vi "DLIbufferedRead.vi"(9 "timeout(ms)":i32, 10 "Ch.":i32, 11 "URL":string) -> (0 "error out":errorcluster, 1 "state(1or0)":i16, 2 "body":string, 3 "headers":string)   [LabVIEW 2018]
uses:
  DLIbufferState.ctl
  ADAM Client/Sub VIs/ADAM Controls/Remember_value_mode.ctl
  <vilib>/httpClient/LabVIEWHTTPClient.lvlib
panel:
  out "AuditTrail":T1[](array[typedef])
  out "allChs":u32 format="%08b"
  out "age(s)":dbl
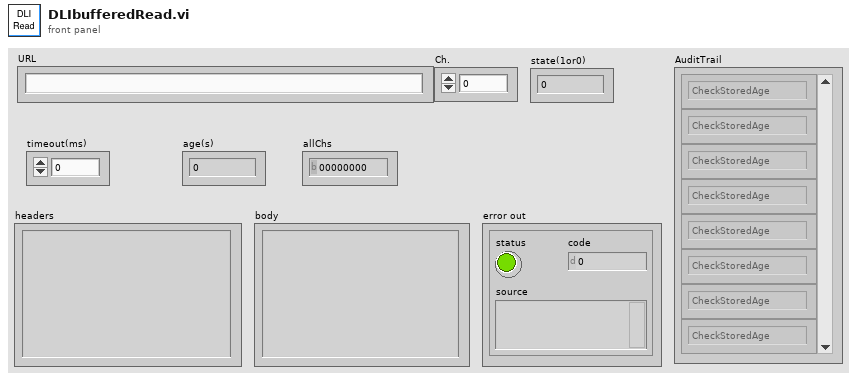
[diagram p1: front panel]
types:
  T1 = typedef "DLIbufferState.ctl" = enum16{"CheckStoredAge", "UseStoredValue", "Read", "Store"}
  T2 = typedef "Remember_value_mode.ctl" = enum16{"Read only", "Read and Write"}
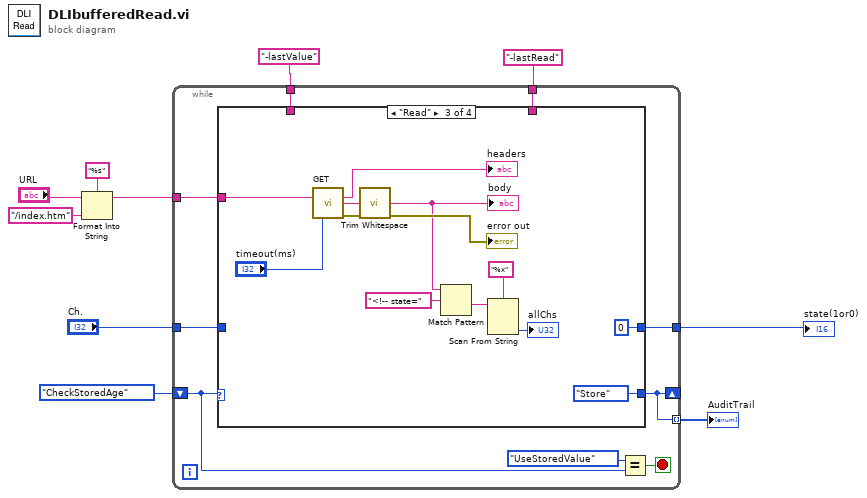
[diagram p0: block diagram]
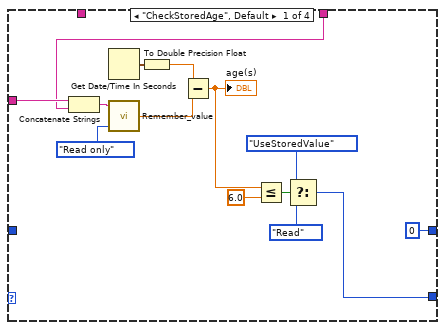
[diagram p2: hidden frame]
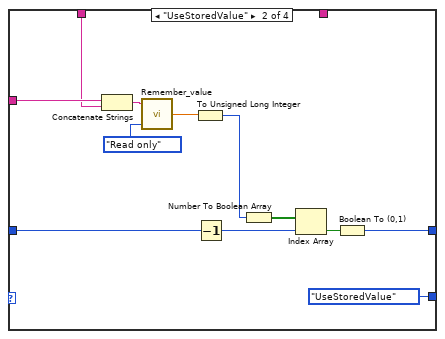
[diagram p3: hidden frame]
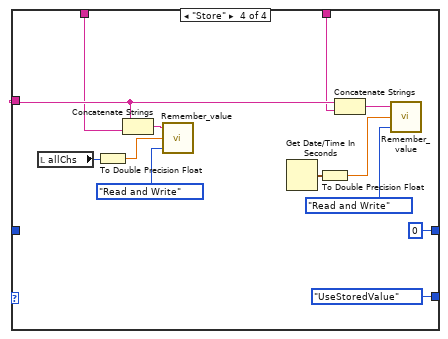
[diagram p4: hidden frame]
diagram:
  n1 = Format Into String(format string="%s", initial string="URL", "/index.htm" ("input 1")) -> (resulting string=w6:string)  [unwired: 1 in, 1 out]
  n2 = while {
    shift-right: [w11] -> _
    shift-left: DLIbufferState."CheckStoredAge" -> [w12]
    tunnel: w6 -> [w19]
    tunnel: "Ch." -> [w18]
    tunnel: [w17] -> w4
    tunnel: "-lastRead" ("string") -> [w16]
    tunnel: "-lastValue" ("string") -> [w15]
    tunnel: [w11] -> w1 mode=indexing
    stop <- w14 stop-if-true
    n3 = case shown="\"Read\"" w12 {
      tunnel: w19 -> [w30 w43 w50 w64]
      tunnel: w18 -> [_ w37 _ _]
      tunnel: [i16 0 w36 i16 0 i16 0] -> w17
      tunnel: [w23 DLIbufferState."UseStoredValue" DLIbufferState."Store" DLIbufferState."UseStoredValue"] -> w11
      tunnel: w16 -> [w20 _ _ w61]
      tunnel: w15 -> [_ w35 _ w60]
      frame "CheckStoredAge", Default {
        n4 = Concatenate Strings(w30, w20) -> (w31:string)
        n5 = Get Date/Time In Seconds() -> (seconds since 1Jan1904=w33:timestamp)
        n6 = call "Remember_value.vi"("Mode"=Remember_value_mode."Read only", "Ch name"=w31) -> ("Output Value"=w28:dbl)  [unwired: 1 in]
        n7 = To Double Precision Float(number=w33) -> (double precision float=w29:dbl)
        n8 = Subtract(x=w29, y=w28) -> (x-y=w27:dbl)
        "age(s)" <- w27
        n9 = Less Or Equal?(x=w27, y=6.0) -> (x <= y?=w25:bool)
        n10 = Select(t=DLIbufferState."UseStoredValue", s=w25, f=DLIbufferState."Read") -> (s? t:f=w23:T1)
      }
      frame "UseStoredValue" {
        n11 = Concatenate Strings(w43, w35) -> (w45:string)
        n12 = call "Remember_value.vi"("Mode"=Remember_value_mode."Read only", "Ch name"=w45) -> ("Output Value"=w39:dbl)  [unwired: 1 in]
        n13 = To Unsigned Long Integer(number=w39) -> (unsigned 32bit integer=w38:u32)
        n14 = Decrement(x=w37) -> (x-1=w41:i32)
        n15 = Number To Boolean Array(number=w38) -> (Boolean array=w40:bool[])
        n16 = Index Array(array=w40, index=w41) -> (element=w42:bool)
        n17 = Boolean To (0,1)(Boolean=w42) -> (0, 1=w36:i16)
      }
      frame "Read" {
        n18 = call <vilib>:"GET.vi"("url"=w50, "timeout (10000)"="timeout(ms)") -> ("headers"=→"headers":string, "body"=w52:string, "error out"=→"error out":errorcluster)  [unwired: 10 in, 1 out]
        n19 = call <vilib>:"Trim Whitespace.vi"("string"=w52) -> ("trimmed string"=w46:string)  [unwired: 1 in]
        "body" <- w46
        n20 = Match Pattern(string=w46, regular expression="<!-- state=") -> (after substring=w56:string)  [unwired: 1 in, 3 out]
        n21 = Scan From String(format string="%x", input string=w56) -> (output 1=→"allChs":u32)  [unwired: 3 in, 3 out]
      }
      frame "Store" {
        n22 = local read "allChs"() -> (w63:u32)
        n23 = To Double Precision Float(number=w63) -> (double precision float=w62:dbl)
        n24 = Concatenate Strings(w64, w60) -> (w70:string)
        n25 = call "Remember_value.vi"("Mode"=Remember_value_mode."Read and Write", "Input Value"=w62, "Ch name"=w70) -> ()  [unwired: 1 out]
        n26 = Get Date/Time In Seconds() -> (seconds since 1Jan1904=w67:timestamp)
        n27 = To Double Precision Float(number=w67) -> (double precision float=w68:dbl)
        n28 = Concatenate Strings(w64, w61) -> (w65:string)
        n29 = call "Remember_value.vi"("Mode"=Remember_value_mode."Read and Write", "Input Value"=w68, "Ch name"=w65) -> ()  [unwired: 1 out]
      }
    }
    n30 = Equal?(x=DLIbufferState."UseStoredValue", y=w12) -> (x = y?=w14:bool)
  }
  "state(1or0)" <- w4
  "AuditTrail" <- w1
